vi "Read Staff Name.vi"(8 "error in (no error)":errorcluster, 11 "Room Service Base in":refnum<class "Room Service Base.lvclass">) -> (0 "error out":errorcluster, 2 "Staff Name":string, 3 "Room Service Base out":refnum<class "Room Service Base.lvclass">)   [LabVIEW 2023, in "Room Service Types.lvlib" / "Room Service Base.lvclass"]
uses:
  Room Service Base.lvclass
  Room Service Base.lvclass/Room Service Base.ctl
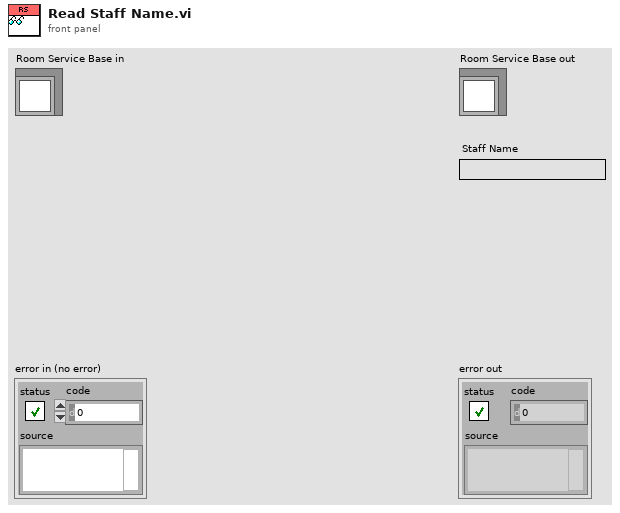
[diagram p1: front panel]
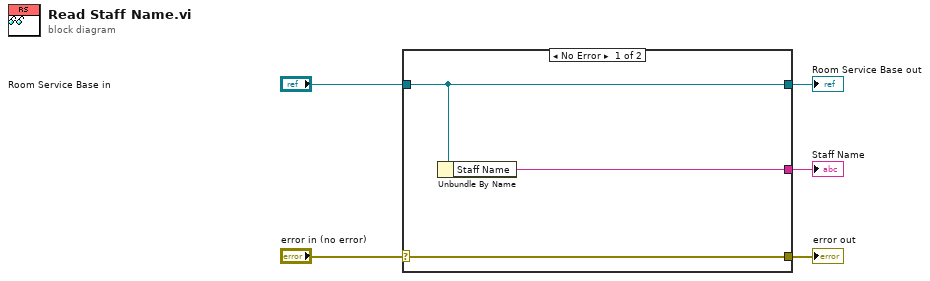
[diagram p0: block diagram]
diagram:
  n1 = case shown="No Error" "error in (no error)" {
    selector: "error in (no error)" -> [w8 w9]
    tunnel: [w8 w9] -> w4
    tunnel: [w7 w10] -> w2
    tunnel: "Room Service Base in" -> [w7 w10]
    tunnel: [w6 _] -> w1
    frame No Error {
      n2 = Unbundle By Name(w7) -> ("Staff Name"=w6:string)
    }
    frame Error {
    }
  }
  "error out" <- w4
  "Room Service Base out" <- w2
  "Staff Name" <- w1
